vi "WriteIO.1.fpga.vi"(10 "x (in)":u32) -> (2 "x (out)":u32)   [LabVIEW 2012]
uses:
  <vilib>/rvi/DataTransferAndStorage/Container/Common/niFpgaContainerGetUniqueNameForEmu.vi
  <vilib>/rvi/Memory/Memory_Emulation/niFpgaMemoryEmulationCacheClearOnFirstRun.vi
  <vilib>/rvi/Memory/Memory_Emulation/nirvimemoryEmulationManagerCache_MakeExclusive.vi
  <vilib>/rvi/Memory/Memory_Emulation/niFpgaMemoryEmulationValidateCache.vi
  <vilib>/rvi/Memory/Memory_Emulation/nirvimemoryEmulationManagerCache_ReleaseExclusive.vi
  <vilib>/rvi/Memory/Memory_Emulation/nirvimemoryEmulationManagerCache_InsertValue.vi
  <vilib>/Utility/error.llb/Clear Errors.vi
  <vilib>/rvi/Memory/Memory_Emulation/nirvimemoryEmulationManagerCache_GetValue.vi
  <vilib>/rvi/eio/common/nirviEmuTemplateMethod_errors.vi
  <vilib>/rvi/DataTransferAndStorage/Container/XNode/niFpgaContainer.xnode
  <vilib>/rvi/Memory/Memory_Emulation/nirvimemoryEmulation.vi
  <vilib>/eio/EIONode/EIONode.xnode
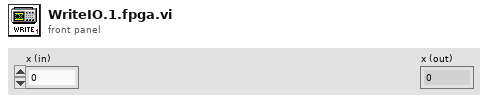
[diagram p1: front panel]
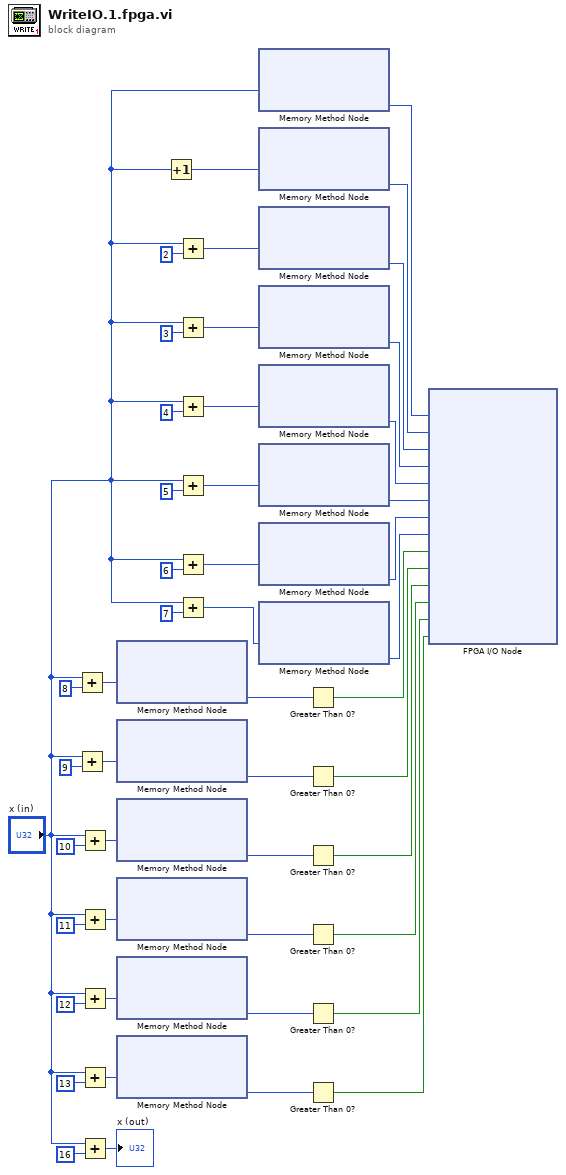
[diagram p0: block diagram]
diagram:
  n1 = Add(x="x (in)", y=u32 8) -> (x+y=w12:u32)
  n2 = Add(x="x (in)", y=u32 9) -> (x+y=w14:u32)
  n3 = Add(x="x (in)", y=u32 10) -> (x+y=w10:u32)
  n4 = Add(x="x (in)", y=u32 11) -> (x+y=w8:u32)
  n5 = Add(x="x (in)", y=u32 12) -> (x+y=w4:u32)
  n6 = Add(x="x (in)", y=u32 13) -> (x+y=w5:u32)
  n7 = Add(x="x (in)", y=u32 16) -> (x+y=→"x (out)":u32)
  n8 = xnode ("Memory Method Node")("Address"=w12) -> ("Data"=w40:i16)  [unwired: 1 in, 1 out]
  n9 = xnode ("Memory Method Node")("Address"=w14) -> ("Data"=w38:i16)  [unwired: 1 in, 1 out]
  n10 = xnode ("Memory Method Node")("Address"=w10) -> ("Data"=w37:i16)  [unwired: 1 in, 1 out]
  n11 = xnode ("Memory Method Node")("Address"=w8) -> ("Data"=w36:i16)  [unwired: 1 in, 1 out]
  n12 = xnode ("Memory Method Node")("Address"=w4) -> ("Data"=w35:i16)  [unwired: 1 in, 1 out]
  n13 = xnode ("Memory Method Node")("Address"=w5) -> ("Data"=w30:i16)  [unwired: 1 in, 1 out]
  n14 = Increment(x="x (in)") -> (x+1=w28:u32)
  n15 = Add(x="x (in)", y=u32 2) -> (x+y=w24:u32)
  n16 = Add(x="x (in)", y=u32 3) -> (x+y=w25:u32)
  n17 = Add(x="x (in)", y=u32 4) -> (x+y=w21:u32)
  n18 = Add(x="x (in)", y=u32 5) -> (x+y=w19:u32)
  n19 = Add(x="x (in)", y=u32 6) -> (x+y=w17:u32)
  n20 = Add(x="x (in)", y=u32 7) -> (x+y=w15:u32)
  n21 = xnode ("Memory Method Node")("Address"="x (in)") -> ("Data"=w48:i16)  [unwired: 1 in, 1 out]
  n22 = xnode ("Memory Method Node")("Address"=w28) -> ("Data"=w47:i16)  [unwired: 1 in, 1 out]
  n23 = xnode ("Memory Method Node")("Address"=w24) -> ("Data"=w46:i16)  [unwired: 1 in, 1 out]
  n24 = xnode ("Memory Method Node")("Address"=w25) -> ("Data"=w45:i16)  [unwired: 1 in, 1 out]
  n25 = xnode ("Memory Method Node")("Address"=w21) -> ("Data"=w44:i16)  [unwired: 1 in, 1 out]
  n26 = xnode ("Memory Method Node")("Address"=w19) -> ("Data"=w43:i16)  [unwired: 1 in, 1 out]
  n27 = xnode ("Memory Method Node")("Address"=w17) -> ("Data"=w42:i16)  [unwired: 1 in, 1 out]
  n28 = xnode ("Memory Method Node")("Address"=w15) -> ("Data"=w41:i16)  [unwired: 1 in, 1 out]
  n29 = Greater Than 0?(x=w40) -> (x > 0?=w39:bool)
  n30 = Greater Than 0?(x=w38) -> (x > 0?=w34:bool)
  n31 = Greater Than 0?(x=w37) -> (x > 0?=w33:bool)
  n32 = Greater Than 0?(x=w36) -> (x > 0?=w32:bool)
  n33 = Greater Than 0?(x=w35) -> (x > 0?=w31:bool)
  n34 = Greater Than 0?(x=w30) -> (x > 0?=w29:bool)
  n35 = xnode "FPGA I/O Node"("Connector0/AO0"=w48, "Connector0/AO1"=w47, "Connector0/AO2"=w46, "Connector0/AO3"=w45, "Connector0/AO4"=w44, "Connector0/AO5"=w43, "Connector0/AO6"=w42, "Connector0/AO7"=w41, "Connector0/DIO0"=w39, "Connector0/DIO1"=w34, "Connector0/DIO2"=w33, "Connector0/DIO3"=w32, "Connector0/DIO4"=w31, "Connector0/DIO5"=w29) -> ()  [unwired: 14 in, 14 out]
